vi "FastPiezoSine.vi"(8 "Sinewave amp (V)":dbl=2000.0 format="%#_6f", 9 "Plateau duration (ms)":dbl=2000.0 format="%#_6f", 10 "Sinewave duration (ms)":dbl=2000.0 format="%#_6f", 11 "Ramp duration (ms)":dbl=2000.0 format="%#_6f") -> (3 "appended array":dbl[](array[numeric]))   [LabVIEW 2016]
panel:
  out "size(s)":i32
  out "Waveform Graph":dbl[](graph)
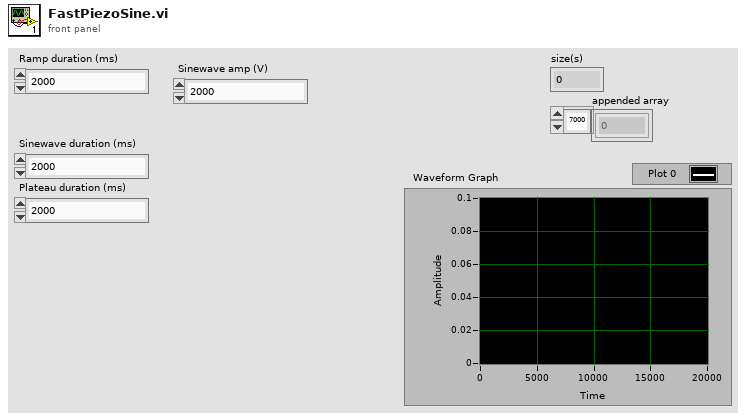
[diagram p1: front panel]
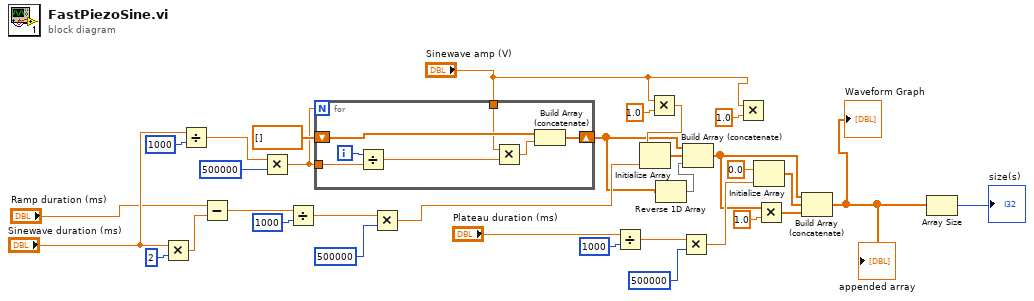
[diagram p0: block diagram]
diagram:
  n1 = Multiply(x="Sinewave duration (ms)", y=2) -> (x*y=w27:dbl)
  n2 = Divide(x="Sinewave duration (ms)", y=1000) -> (x/y=w30:dbl)
  n3 = Subtract(x="Ramp duration (ms)", y=w27) -> (x-y=w21:dbl)
  n4 = Multiply(x=w30, y=500000) -> (x*y=w29:dbl)
  n5 = Divide(x=w21, y=1000) -> (x/y=w22:dbl)
  n6 = for {
    N: w29 -> [_]
    shift-right: [w40] -> w2
    shift-left: dbl[] [] -> [w39]
    tunnel: w29 -> [w38]
    tunnel: "Sinewave amp (V)" -> [w36]
    i -> [w37]
    n7 = Divide(x=w37, y=w38) -> (x/y=w34:dbl)
    n8 = Multiply(x=w36, y=w34) -> (x*y=w35:dbl)
    n9 = Build Array (concatenate)(w39, w35) -> (w40:dbl[])
  }
  n10 = Multiply(x=w22, y=500000) -> (x*y=w20:dbl)
  n11 = Divide(x="Plateau duration (ms)", y=1000) -> (x/y=w17:dbl)
  n12 = Multiply(x="Sinewave amp (V)", y=1.0) -> (x*y=w7:dbl)
  n13 = Initialize Array(w7, w20) -> (w4:dbl[])
  n14 = Reverse 1D Array(array=w2) -> (reversed array=w6:dbl[])
  n15 = Multiply(x=w17, y=500000) -> (x*y=w15:dbl)
  n16 = Build Array (concatenate)(w2, w4, w6) -> (w3:dbl[])
  n17 = Multiply(x="Sinewave amp (V)", y=1.0) -> ()  [unwired: 1 out]
  n18 = Initialize Array(0.0 ("element"), w15) -> (w14:dbl[])
  n19 = Multiply(x=w3, y=1.0) -> (x*y=w12:dbl[])
  n20 = Build Array (concatenate)(w3, w14, w12) -> (w1:dbl[])
  "Waveform Graph" <- w1
  "appended array" <- w1
  n21 = Array Size(array=w1) -> (size(s)=→"size(s)":i32)
